vi "main.vi"() -> ()   [LabVIEW 2011]
uses:
  <vilib>/userdefined/High Color/IMAQdx.ctl
  global_vars.vi
  <userlib>/_OpenG.lib/file/file.llb/Build Path - Traditional__ogtk.vi
  <vilib>/vision/NI_Vision_Development_Module.lvlib
  <vilib>/vision/driver/NI_Vision_Acquisition_Software.lvlib
panel:
  in  "b_record images":bool
  in  "save phasemap":bool
  out "ul_ar_pxar_capt_image":u8[][][](array[numeric])
  out "ul_ar_pxar_orig_patterns":u8[][][](array[numeric])
  in  "Color":u32(colorbox)=16448250
  out "ID_camera in use":T1="HP Webcam"
  in  "UL_#Phase Shifts":i32=4
  out "p_experiment_path":path
  in  "EXP File Path 2":path=path "X:/Cloud Drives/Dropbox/Europhotonics/FringeMan/Image Storage" caption="Enter or select file path"
  in  "save images":bool
  in  "start \nmeasurement":bool
  in  "center radius":dbl
  in  "Alignment":bool=TRUE
  in  "number of rings":i32=20
  in  "flip direction":bool
  in  "fringe/stripe":bool=TRUE
  in  "line position (rel)":i32(slide) min=0 max=100 scale=0.0..100.0
  in  "df_#fringes":dbl=4.0 caption="#fringes"
  in  "fullscreen?":bool
  in  "to second screen":bool
  in  "floating":bool=TRUE
  in  "title bar":bool=TRUE
  in  "y height(Px)":i32=500
  in  "x Width(Px)":i32=1000
  in  "Stop Button":bool
  # "Window Control"
  # "Line & Fringe Control"
  # "Alignment Control"
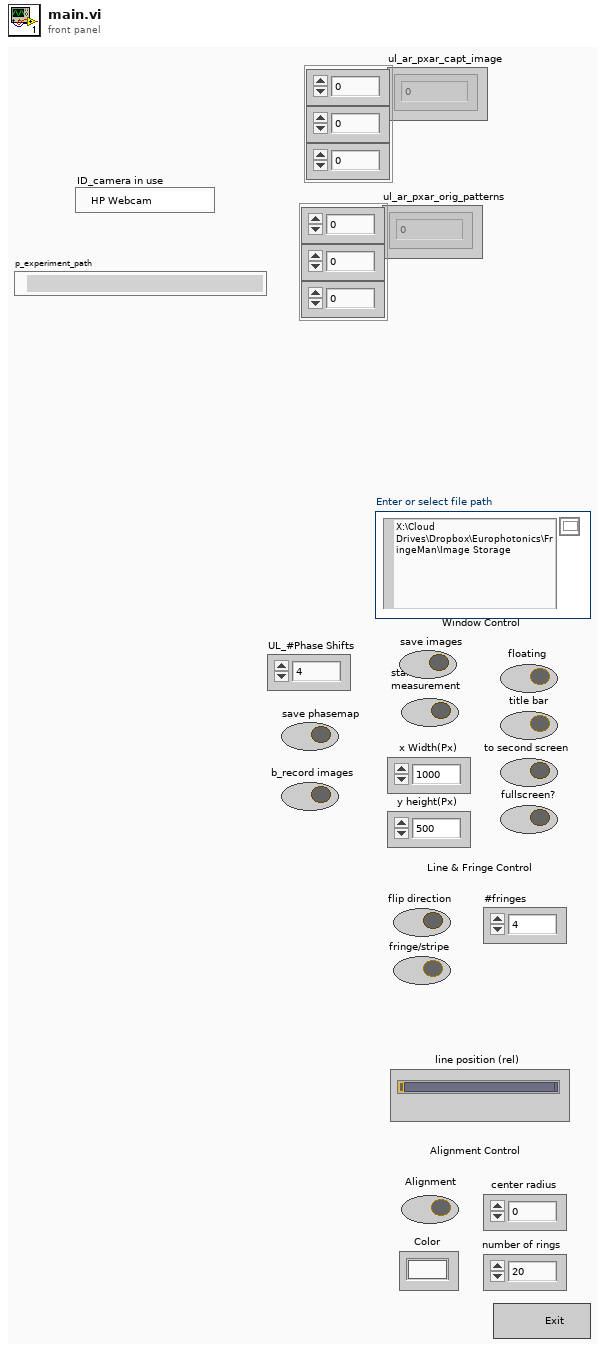
[diagram p1: front panel]
types:
  T1 = typedef "IMAQdx.ctl" = refnum<k21>
  T2 = cluster{"Numeric Control":i16, "Numeric Control":i16}
  T3 = typedef "IMAQ Image.ctl" = refnum<image>
  T4 = typedef "Image Type" = u32
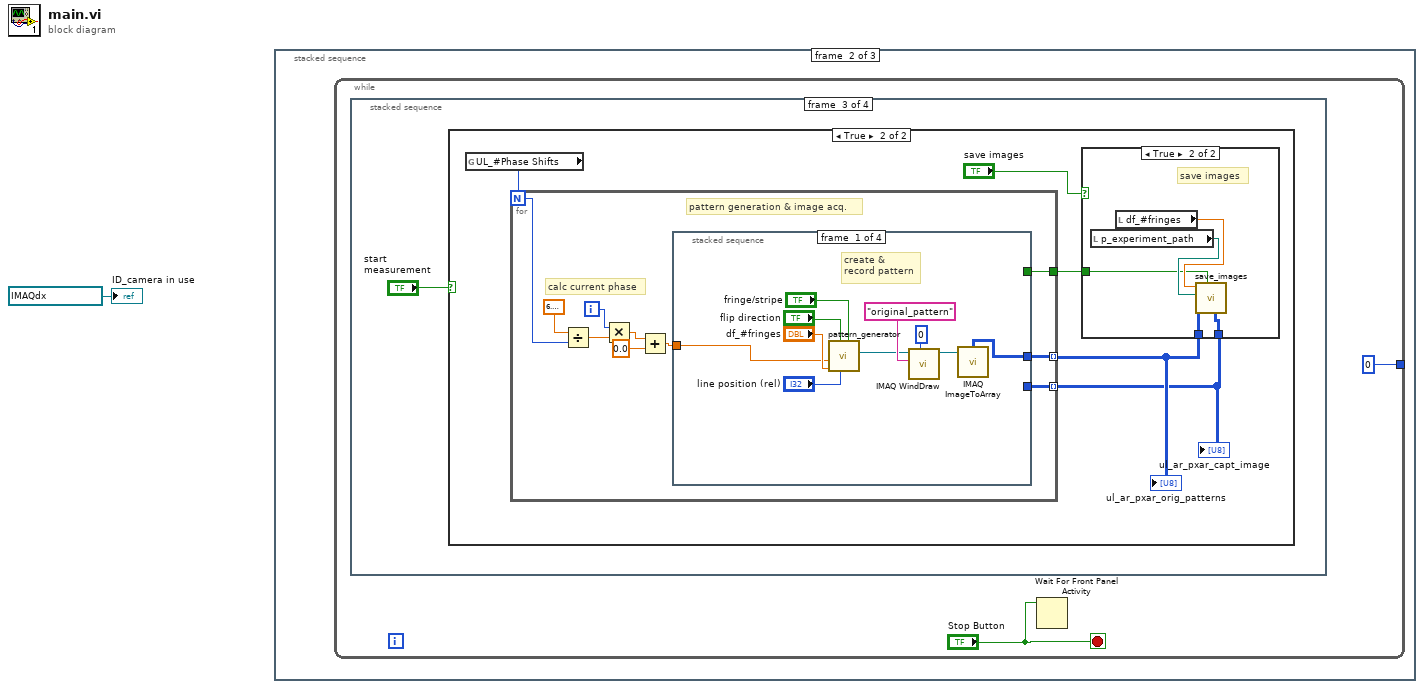
[diagram p0: block diagram]
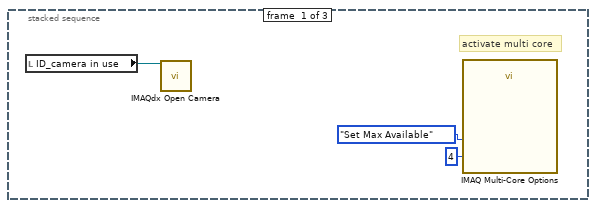
[diagram p2: hidden frame]
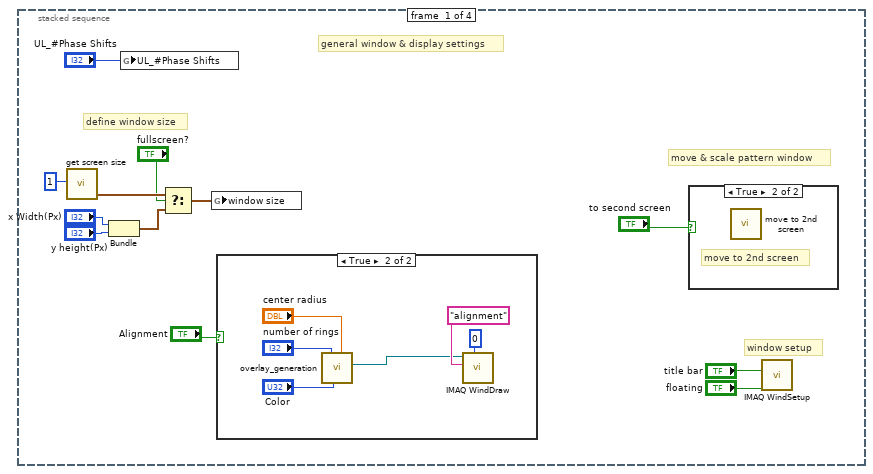
[diagram p3: hidden frame]
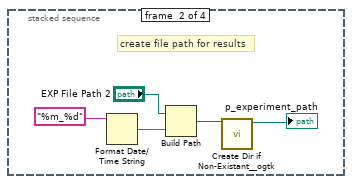
[diagram p6: hidden frame]
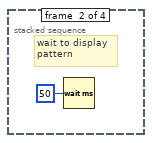
[diagram p9: hidden frame]
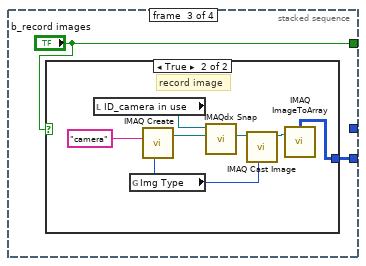
[diagram p10: hidden frame]
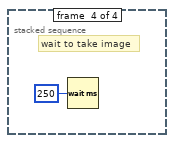
[diagram p12: hidden frame]
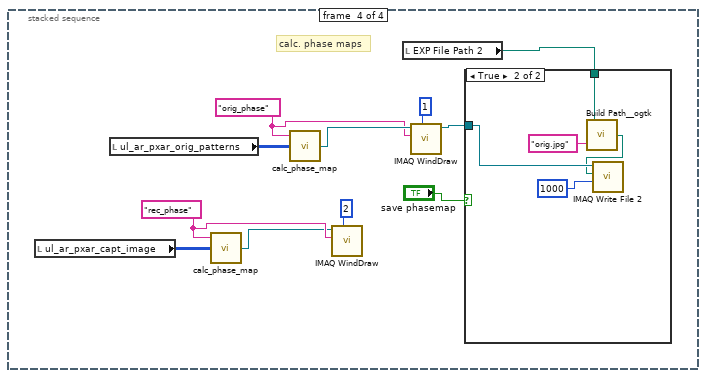
[diagram p13: hidden frame]
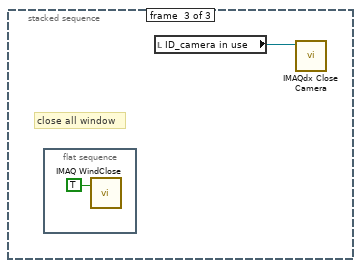
[diagram p15: hidden frame]
diagram:
  n1 = stacked-sequence {
    frame #0 {
      # "activate multi core"
      n2 = local read "ID_camera in use"() -> (w2:T1)
      n3 = call <vilib>:"IMAQdx Open Camera.vi"("Session In"=w2) -> ()  [unwired: 9 in, 2 out]
      n4 = call "IMAQ Multi-Core Options"("Get/Set Number of Cores (Get)"=enum32{"Get", "Set", "Set Max Available"}."Set Max Available", "Specified Number of Cores"=u32 4) -> ()  [unwired: 8 in, 2 out]
    }
    frame #1 {
      n5 = while {
        tunnel: [0] -> _
        stop <- "Stop Button" stop-if-true
        n6 = stacked-sequence {
          frame #0 {
            # "general window & display settings"
            # "define window size"
            # "window setup"
            # "move & scale pattern window"
            n7 = call "get screen size.vi"("screen"=1) -> ("wind size (width/height)"=w12:T2)  [unwired: 2 in, 2 out]
            n8 = Bundle("x Width(Px)"="x Width(Px)", "y height(Px)"="y height(Px)") -> (w10:cluster{"x Width(Px)":i32, "y height(Px)":i32})  [unwired: 1 in]
            n9 = global write "global_vars.vi" "UL_#Phase Shifts"("UL_#Phase Shifts") -> ()
            n10 = Select(t=w12, s="fullscreen?", f=w10) -> (s? t:f=w9:cluster{"x Width(Px)":i32, "y height(Px)":i32})
            n11 = global write "global_vars.vi" "window size"(w9) -> ()
            n12 = case shown="True" "Alignment" {
              frame False {
              }
              frame True {
                n13 = call "overlay_generation.vi"("center radius"="center radius", "Color"="Color", "number of rings"="number of rings") -> ("Image Out"=w20:T3)  [unwired: 8 in]
                n14 = call "IMAQ WindDraw"("Window Number (0...15)"=0, "Title"="alignment", "Image"=w20) -> ()  [unwired: 7 in, 2 out]
              }
            }
            n15 = case shown="True" "to second screen" {
              frame False {
              }
              frame True {
                # "move to 2nd screen"
                n16 = call "move to 2nd screen.vi"() -> ()  [unwired: 12 in]
              }
            }
            n17 = call "IMAQ WindSetup"("Window is floating? (No)"="floating", "Window has title bar? (Yes)"="title bar") -> ()  [unwired: 9 in, 1 out]
          }
          frame #1 {
            # "create file path for results"
            n18 = Format Date/Time String(time format string (%c)="%m_%d") -> (date/time string=w27:string)  [unwired: 2 in]
            n19 = Build Path(base path="EXP File Path 2", name or relative path=w27) -> (appended path=w26:path)
            n20 = call <userlib>:"Create Dir if Non-Existant__ogtk.vi"("Directory Path"=w26) -> ("dup Directory Path"=→"p_experiment_path":path)  [unwired: 8 in, 2 out]
          }
          frame #2 {
            n21 = case shown="True" "start \nmeasurement" {
              frame False {
              }
              frame True {
                n22 = global read "global_vars.vi" "UL_#Phase Shifts"() -> (w35:i32)
                n23 = for {
                  N: w35 -> [w46]
                  tunnel: [w44] -> w34 mode=indexing
                  tunnel: [w42] -> w33 mode=indexing
                  tunnel: [w43] -> w31
                  i -> [w45]
                  # "calc current phase"
                  # "pattern generation & image acq."
                  n24 = Divide(x=6.283185307179586, y=w46) -> (x/y=w49:dbl)
                  n25 = Multiply(x=w45, y=w49) -> (x*y=w48:dbl)
                  n26 = Add(x=w48, y=0.0) -> (x+y=w47:dbl)
                  n27 = stacked-sequence {
                    tunnel: w47 -> [w53 _ _ _]
                    tunnel: [w51 _ _ _] -> w44
                    tunnel: [_ _ "b_record images" _] -> w43
                    tunnel: [_ _ w62 _] -> w42
                    frame #0 {
                      # "create & \nrecord pattern"
                      n28 = call "pattern_generator.vi"("fringe/stripe"="fringe/stripe", "line position (px)"="line position (rel)", "flip direction"="flip direction", "fringe number"="df_#fringes", "phase"=w53) -> ("fringe pattern"=w54:T3)  [unwired: 5 in, 1 out]
                      n29 = call "IMAQ WindDraw"("Window Number (0...15)"=0, "Title"="original_pattern", "Image"=w54) -> ("Image Out (duplicate)"=w52:T3)  [unwired: 7 in, 1 out]
                      n30 = call "IMAQ ImageToArray"("Image"=w52) -> ("Image Pixels (U8)"=w51:u8[][])  [unwired: 3 in, 4 out]
                    }
                    frame #1 {
                      # "wait to display \npattern"
                      n31 = Wait (ms)(milliseconds to wait=u32 50) -> ()  [unwired: 1 out]
                    }
                    frame #2 {
                      n32 = case shown="True" "b_record images" {
                        tunnel: [_ w64] -> w62
                        frame False {
                        }
                        frame True {
                          # "record image"
                          n33 = local read "ID_camera in use"() -> (w68:T1)
                          n34 = global read "global_vars.vi" "Img Type"() -> (w65:T4)
                          n35 = call "IMAQ Create"("Image Name"="camera", "Image Type"=w65) -> ("New Image"=w70:T3)  [unwired: 2 in, 2 out]
                          n36 = call <vilib>:"IMAQdx Snap.vi"("Image In"=w70, "Session In"=w68) -> ("Image Out"=w67:T3)  [unwired: 7 in, 2 out]
                          n37 = call "IMAQ Cast Image"("Image Type"=w65, "Image Src"=w67) -> ("Image Dst Out"=w66:T3)  [unwired: 8 in, 1 out]
                          n38 = call "IMAQ ImageToArray"("Image"=w66) -> ("Image Pixels (U8)"=w64:u8[][])  [unwired: 3 in, 4 out]
                        }
                      }
                    }
                    frame #3 {
                      # "wait to take image"
                      n39 = Wait (ms)(milliseconds to wait=u32 250) -> ()  [unwired: 1 out]
                    }
                  }
                }
                "ul_ar_pxar_orig_patterns" <- w34
                "ul_ar_pxar_capt_image" <- w33
                n40 = case shown="True" "save images" {
                  tunnel: w34 -> [_ w38]
                  tunnel: w33 -> [_ w39]
                  tunnel: w31 -> [_ w36]
                  frame False {
                  }
                  frame True {
                    # "save images"
                    n41 = local read "p_experiment_path"() -> (w37:path)
                    n42 = local read "df_#fringes"() -> (w40:dbl)
                    n43 = call "save_images.vi"("ul_ar_pxar_capt_image"=w39, "ul_ar_pxar_orig_pattern"=w38, "save recorded images"=w36, "p_experiment_path"=w37, "number of fringes"=w40) -> ()  [unwired: 7 in]
                  }
                }
              }
            }
          }
          frame #3 {
            w76 = "rec_phase" ("String")
            w77 = "orig_phase" ("String")
            # "calc. phase maps"
            n44 = local read "ul_ar_pxar_capt_image"() -> (w73:u8[][][])
            n45 = local read "ul_ar_pxar_orig_patterns"() -> (w82:u8[][][])
            n46 = call "calc_phase_map.vi"("u8_ar_image_pixel_array"=w73, "image name"=w76) -> ("phase map"=w75:T3)  [unwired: 2 in, 1 out]
            n47 = call "calc_phase_map.vi"("u8_ar_image_pixel_array"=w82, "image name"=w77) -> ("phase map"=w80:T3)  [unwired: 2 in, 1 out]
            n48 = call "IMAQ WindDraw"("Window Number (0...15)"=2, "Title"=w76, "Image"=w75) -> ()  [unwired: 7 in, 2 out]
            n49 = local read "EXP File Path 2"() -> (w78:path)
            n50 = call "IMAQ WindDraw"("Window Number (0...15)"=1, "Title"=w77, "Image"=w80) -> ("Image Out (duplicate)"=w79:T3)  [unwired: 7 in, 1 out]
            n51 = case shown="True" "save phasemap" {
              tunnel: w79 -> [_ w87]
              tunnel: w78 -> [_ w83]
              frame False {
              }
              frame True {
                n52 = call-poly <userlib>:"Build Path__ogtk.vi"("name or relative path"="orig.jpg", "base path"=w83) -> ("appended path"=w84:path)
                n53 = call-poly "IMAQ Write File 2"("Image Quality"=u32 1000, "File Path"=w84, "Image"=w87) -> ()  [unwired: 7 in, 2 out]
              }
            }
          }
        }
        n54 = Wait For Front Panel Activity(3:"Stop Button") -> ()  [unwired: 2 in, 1 out]
      }
    }
    frame #2 {
      # "close all window"
      n55 = flat-sequence {
        frame #0 {
          n56 = call "IMAQ WindClose"("Close All Windows (False)"=TRUE) -> ()  [unwired: 5 in, 1 out]
        }
      }
      n57 = local read "ID_camera in use"() -> (w88:T1)
      n58 = call <vilib>:"IMAQdx Close Camera.vi"("Session In"=w88) -> ()  [unwired: 10 in, 1 out]
    }
  }
  "ID_camera in use" <- T1 "HP Webcam" ("Session In")
